vi "Migrate Common Dependencies.vi"(0 "Project path":path, 5 "Measurement path":path, 7 "Dependencies path":path[](array[path]), 11 "error in (no error)":errorcluster) -> (4 "Project reference":refnum<vi>, 6 "MeasurementCore reference":refnum<vi>, 8 "Outside items":string[](array[string]), 15 "error out":errorcluster)   [LabVIEW 2021]
uses:
  controls/Library Info.ctl
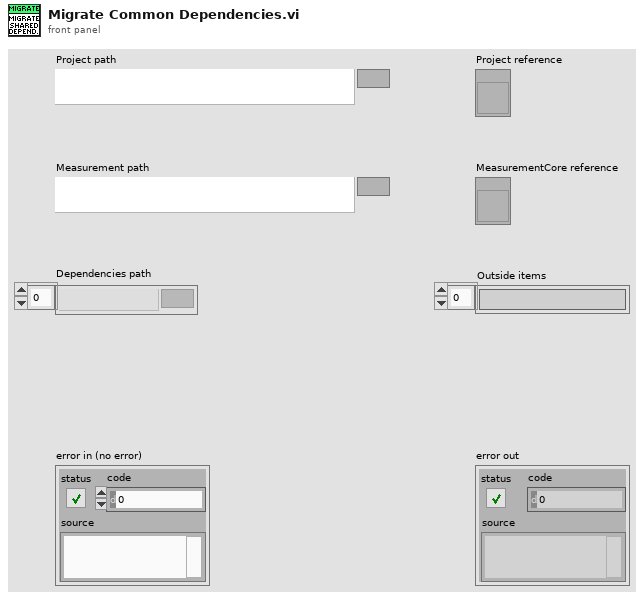
[diagram p1: front panel]
types:
  T1 = typedef "Library Info.ctl" = cluster{"Library path":path, "Library name":string}
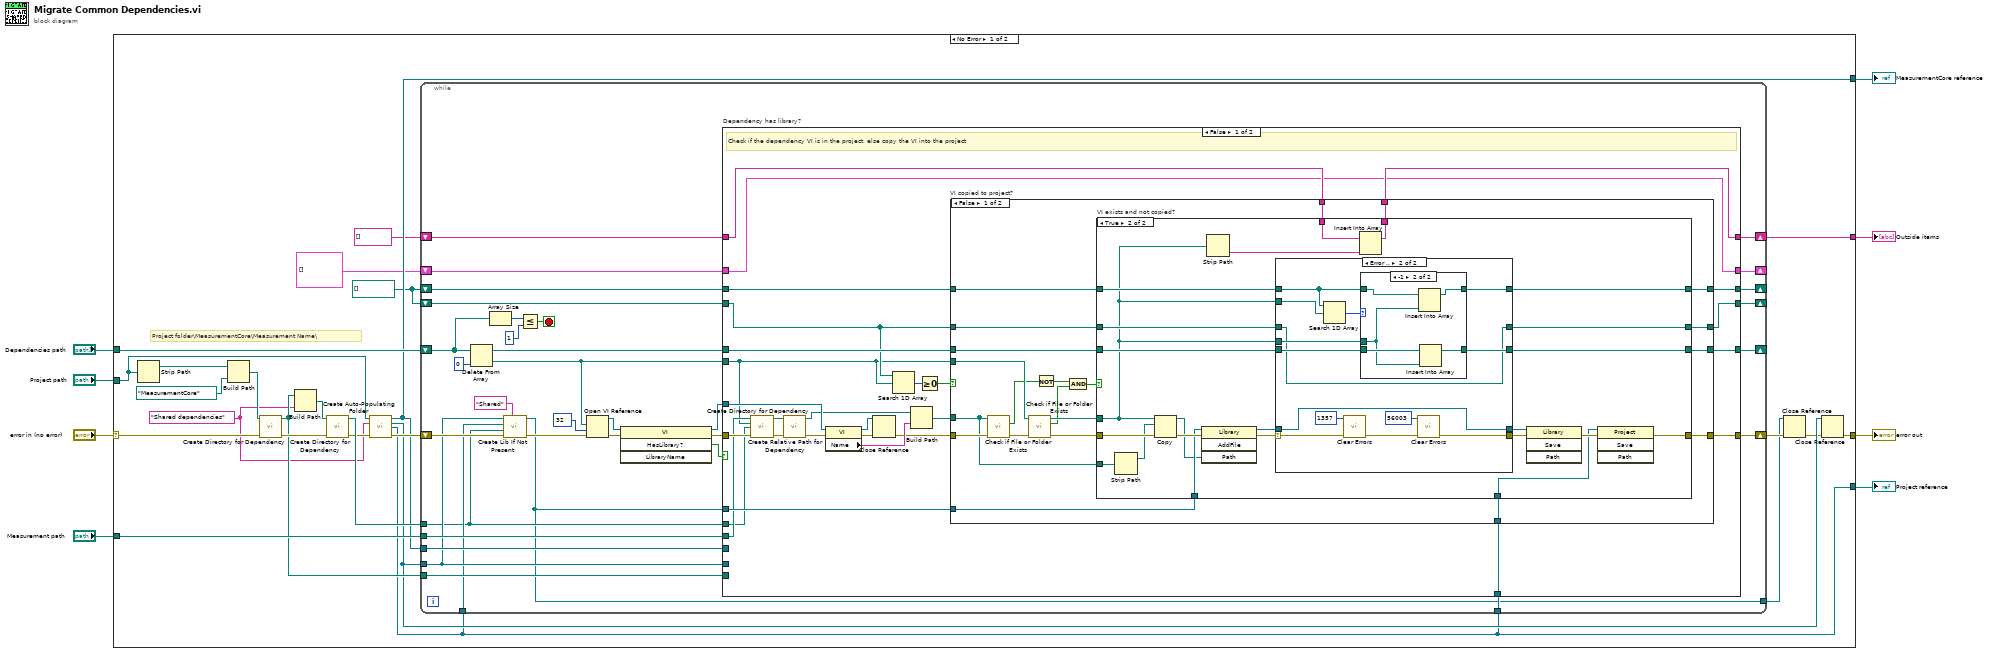
[diagram p0: block diagram]
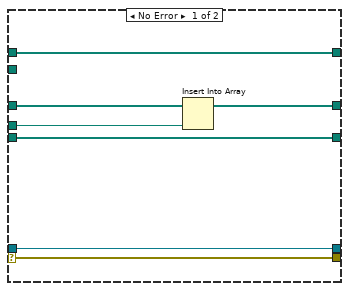
[diagram p3: hidden frame]
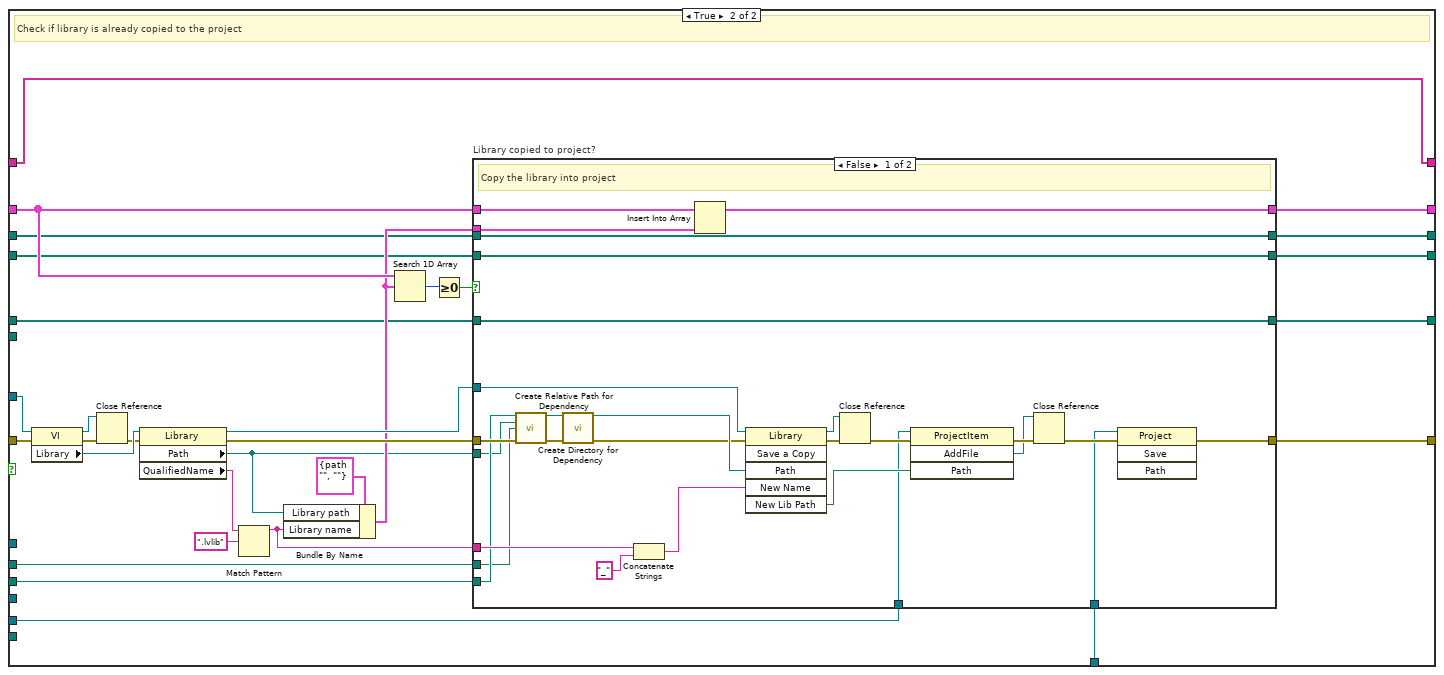
[diagram p6: hidden frame]
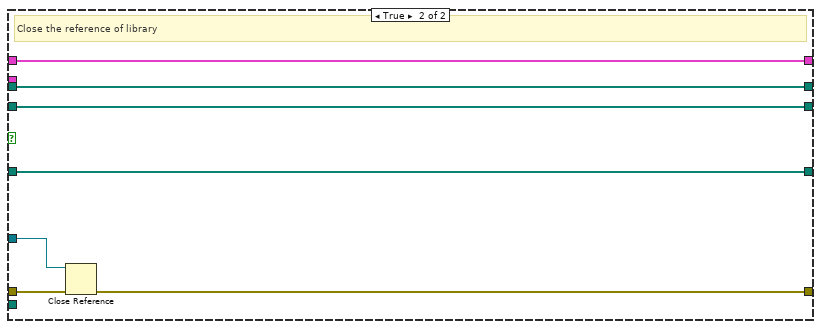
[diagram p7: hidden frame]
diagram:
  n1 = case shown="No Error" "error in (no error)" {
    selector: "error in (no error)" -> [w25 w243]
    tunnel: [w18 w243] -> w7
    tunnel: "Project path" -> [w24 _]
    tunnel: "Measurement path" -> [w29 _]
    tunnel: "Dependencies path" -> [w33 _]
    tunnel: [w20 _] -> w3
    tunnel: [w14 _] -> w2
    tunnel: [w15 _] -> w1
    frame No Error {
      w10 = "Shared dependencies"
      w11 = path[] []
      # "Project folder\\MeasurementCore\\Measurement Name\\"
      n2 = Strip Path(path=w24) -> (stripped path=w28:path)  [unwired: 1 out]
      n3 = Build Path(base path=w28, name or relative path=path "MeasurementCore") -> (appended path=w26:path)
      n4 = call "Create Directory for Dependency.vi"("Directory path"=w26, "error in (no error)"=w25) -> ("Directory path out"=w19:path, "error out"=w23:errorcluster)  [unwired: 12 in]
      n5 = Build Path(base path=w19, name or relative path=w10) -> (appended path=w32:path)
      n6 = call "Create Directory for Dependency.vi"("Directory path"=w32, "error in (no error)"=w23) -> ("Directory path out"=w31:path, "error out"=w22:errorcluster)  [unwired: 12 in]
      n7 = call "Create Auto-Populating Folder.vi"("Project path"=w24, "Plug-in name"=w10, "error in (no error)"=w22) -> ("MeasurementCore reference"=w20:refnum<vi>, "Folder reference"=w17:refnum<vi>, "Project reference"=w14:refnum<vi>, "error out"=w21:errorcluster)  [unwired: 9 in]
      n8 = while {
        shift-right: [w55] -> w30
        shift-left: w21 -> [w43]
        shift-right: [w48] -> _
        shift-left: w33 -> [w65]
        tunnel: w31 -> [w39]
        shift-right: [w54] -> _
        shift-left: T1[] [] -> [w57]
        tunnel: w29 -> [w53]
        shift-right: [w50] -> _
        shift-left: w11 -> [w51]
        tunnel: w20 -> [w47]
        tunnel: w19 -> [w46]
        tunnel: w17 -> [w41]
        shift-right: [w44] -> w15
        shift-left: string[] [] -> [w45]
        tunnel: w14 -> [w40]
        tunnel: w14 -> [w38]
        shift-right: [w37] -> _
        shift-left: w11 -> [w36]
        tunnel: [w35] -> w12
        stop <- w64 stop-if-true
        n9 = Delete From Array(array=w65, index=0) -> (deleted portion=w52:path, array with subset deleted=w49:path[])  [unwired: 1 in]
        n10 = Array Size(array=w65) -> (size(s)=w67:i32)
        n11 = call "Create Lib If Not Present.vi"("Plug-in name"="Shared", "error in (no error)"=w43, "DestDirectory"=w39, "ProjectRef"=w40, "VirtualFolderRef"=w41) -> ("error out"=w42:errorcluster, "Library Refnum"=w35:refnum<vi>)  [unwired: 5 in]
        n12 = Less Or Equal?(x=w67, y=1) -> (x <= y?=w64:bool)
        n13 = Open VI Reference(vi path=w52, options=32, error in (no error)=w42) -> (vi reference=w61:refnum<vi>, error out=w63:errorcluster)  [unwired: 3 in]
        n14 = invoke class="VI" method="HasLibrary?"(reference=w61, error in=w63) -> (reference out=w58:refnum<vi>, error out=w59:errorcluster, "Has Library?"=w60:bool)  [unwired: 2 in, 1 out]
        n15 = case "Dependency has library?" shown="False" w60 {
          tunnel: w59 -> [w73 w206]
          tunnel: w58 -> [w94 w207]
          tunnel: w57 -> [w77 w194]
          tunnel: [w89 w195] -> w55
          tunnel: [w77 w193] -> w54
          tunnel: w53 -> [w72 w191]
          tunnel: w39 -> [w70 w189]
          tunnel: w52 -> [w71 _]
          tunnel: w51 -> [w85 w186]
          tunnel: [w81 w185] -> w50
          tunnel: w49 -> [w88 w184]
          tunnel: [w87 w183] -> w48
          tunnel: w47 -> [_ _]
          tunnel: w46 -> [_ _]
          tunnel: w41 -> [_ w182]
          tunnel: w45 -> [w79 w181]
          tunnel: [w78 w181] -> w44
          tunnel: w35 -> [w80 _]
          tunnel: w38 -> [w74 w180]
          tunnel: [w76 w178] -> w37
          tunnel: w36 -> [w75 w179]
          frame False {
            # "Check if the dependency VI is in the project, else copy the VI into the project"
            n16 = call "Create Relative Path for Dependency.vi"("Old Main Path"=w72, "Old Dependency Path"=w71, "New Dir"=w70, "error in (no error)"=w73) -> ("Directory"=w68:path, "error out"=w69:errorcluster)  [unwired: 10 in]
            n17 = call "Create Directory for Dependency.vi"("Directory path"=w68, "error in (no error)"=w69) -> ("Directory path out"=w86:path, "error out"=w95:errorcluster)  [unwired: 12 in]
            n18 = property class="VI"(reference=w94, error in=w95) -> (reference out=w90:refnum<vi>, error out=w93:errorcluster, "Name"=w92:string)
            n19 = Close Reference(reference=w90, error in (no error)=w93) -> (error out=w91:errorcluster)
            n20 = Search 1D Array(1D array=w85, element=w71) -> (index of element=w84:i32)  [unwired: 1 in]
            n21 = Build Path(base path=w86, name or relative path=w92) -> (appended path=w83:path)
            n22 = Greater Or Equal To 0?(x=w84) -> (x >= 0?=w82:bool)
            n23 = case "VI copied to project?" shown="False" w82 {
              tunnel: w91 -> [w116 w177]
              tunnel: w71 -> [w115 _]
              tunnel: [w112 w177] -> w89
              tunnel: w85 -> [w111 w176]
              tunnel: [w110 w176] -> w81
              tunnel: w83 -> [w106 _]
              tunnel: w88 -> [w109 w175]
              tunnel: [w108 w175] -> w87
              tunnel: w79 -> [w101 w174]
              tunnel: [w100 w174] -> w78
              tunnel: w80 -> [w99 _]
              tunnel: [w98 w173] -> w76
              tunnel: w75 -> [w97 w173]
              tunnel: w74 -> [w96 _]
              frame False {
                n24 = call <vilib>:"Check if File or Folder Exists.vi"("error in (no error)"=w116, "path"=w106) -> ("error out"=w107:errorcluster, "file or folder exists?"=w105:bool)  [unwired: 7 in, 1 out]
                n25 = call <vilib>:"Check if File or Folder Exists.vi"("error in (no error)"=w107, "path"=w115) -> ("error out"=w114:errorcluster, "file or folder exists?"=w103:bool, "dup path"=w113:path)  [unwired: 7 in]
                n26 = Not(x=w105) -> (.not. x?=w104:bool)
                n27 = And(x=w104, y=w103) -> (x .and. y?=w102:bool)
                n28 = case "VI exists and not copied?" shown="True" w102 {
                  tunnel: w114 -> [w121 w144]
                  tunnel: w113 -> [_ w122]
                  tunnel: [w121 w124] -> w112
                  tunnel: w111 -> [w120 w143]
                  tunnel: [w120 w142] -> w110
                  tunnel: w106 -> [_ w138]
                  tunnel: w109 -> [w119 w126]
                  tunnel: [w119 w125] -> w108
                  tunnel: w101 -> [w118 w137]
                  tunnel: [w118 w135] -> w100
                  tunnel: w99 -> [_ w134]
                  tunnel: [w117 w132] -> w98
                  tunnel: w97 -> [w117 w131]
                  tunnel: w96 -> [_ w123]
                  frame False {
                  }
                  frame True {
                    n29 = Strip Path(path=w138) -> (stripped path=w140:path)  [unwired: 1 out]
                    n30 = Copy(8:w144, 10:w140, 11:w122) -> (0:w141:errorcluster, 3:w133:path)  [unwired: 2 in, 1 out]
                    n31 = invoke class="Library" method="AddFile"(reference=w134, error in=w141, "Path"=w133) -> (reference out=w130:refnum<vi>, error out=w129:errorcluster)  [unwired: 1 in, 2 out]
                    n32 = Strip Path(path=w122) -> (name=w136:string)  [unwired: 1 out]
                    n33 = case shown="Error .." w129 {
                      selector: w129 -> [w146 w165]
                      tunnel: w143 -> [w151 w152]
                      tunnel: [w150 w152] -> w142
                      tunnel: w122 -> [w149 w155]
                      tunnel: [w148 w156] -> w132
                      tunnel: w131 -> [w148 w157]
                      tunnel: [w147 w154] -> w127
                      tunnel: w130 -> [w147 w154]
                      tunnel: [w146 w163] -> w128
                      tunnel: w126 -> [w145 w159]
                      tunnel: [w145 w158] -> w125
                      tunnel: w122 -> [_ w160]
                      frame No Error {
                        n34 = Insert Into Array(array=w151, new element=w149) -> (w150:path[])  [unwired: 1 in]
                      }
                      frame Error {
                        n35 = Search 1D Array(1D array=w157, element=w160) -> (index of element=w153:i32)  [unwired: 1 in]
                        n36 = call <vilib>:"Clear Errors.vi"("error in (no error)"=w165, "specific error code to clear (0: all)"=1357) -> ("error out"=w164:errorcluster)  [unwired: 4 in, 1 out]
                        n37 = case shown="-1" w153 {
                          tunnel: w159 -> [w166 w172]
                          tunnel: [w166 w171] -> w158
                          tunnel: w157 -> [w167 w170]
                          tunnel: [w167 w169] -> w156
                          tunnel: w155 -> [_ w168]
                          frame Default {
                          }
                          frame -1 {
                            n38 = Insert Into Array(array=w170, new element=w168) -> (w169:path[])  [unwired: 1 in]
                            n39 = Insert Into Array(array=w172, new element=w168) -> (w171:path[])  [unwired: 1 in]
                          }
                        }
                        n40 = call <vilib>:"Clear Errors.vi"("error in (no error)"=w164, "specific error code to clear (0: all)"=56003) -> ("error out"=w163:errorcluster)  [unwired: 4 in, 1 out]
                      }
                    }
                    n41 = Insert Into Array(array=w137, new element=w136) -> (w135:string[])  [unwired: 1 in]
                    n42 = invoke class="Library" method="Save"(reference=w127, error in=w128) -> (error out=w139:errorcluster)  [unwired: 2 in, 3 out]
                    n43 = invoke class="Project" method="Save"(reference=w123, error in=w139) -> (error out=w124:errorcluster)  [unwired: 2 in, 3 out]
                  }
                }
              }
              frame True {
              }
            }
          }
          frame True {
            # "Check if library is already copied to the project"
            n44 = property class="VI"(reference=w207, error in=w206) -> (reference out=w197:refnum<vi>, error out=w205:errorcluster, "Library"=w204:refnum<vi>)
            n45 = Close Reference(reference=w197, error in (no error)=w205) -> (error out=w198:errorcluster)
            n46 = property class="Library"(reference=w204, error in=w198) -> (reference out=w196:refnum<vi>, error out=w199:errorcluster, "Path"=w190:path, "QualifiedName"=w200:string)
            n47 = Match Pattern(string=w200, regular expression=".lvlib") -> (before substring=w187:string)  [unwired: 1 in, 3 out]
            n48 = Bundle By Name(cluster=T1 {"Library path"=path "", "Library name"=""} ("Cluster"), "Library path"=w190, "Library name"=w187) -> (w192:T1)
            n49 = Search 1D Array(1D array=w194, element=w192) -> (index of element=w202:i32)  [unwired: 1 in]
            n50 = Greater Or Equal To 0?(x=w202) -> (x >= 0?=w201:bool)
            n51 = case "Library copied to project?" shown="False" w201 {
              tunnel: w199 -> [w212 w241]
              tunnel: w196 -> [w229 w242]
              tunnel: [w216 w240] -> w195
              tunnel: w194 -> [w235 w239]
              tunnel: [w234 w239] -> w193
              tunnel: w192 -> [w233 _]
              tunnel: w191 -> [w211 _]
              tunnel: w190 -> [w210 _]
              tunnel: w189 -> [w209 _]
              tunnel: w187 -> [w219 _]
              tunnel: w186 -> [w226 w238]
              tunnel: [w226 w238] -> w185
              tunnel: [w225 w237] -> w183
              tunnel: w184 -> [w225 w237]
              tunnel: w182 -> [w220 _]
              tunnel: w180 -> [w215 _]
              tunnel: [w214 w236] -> w178
              tunnel: w179 -> [w214 w236]
              frame False {
                # "Copy the library into project"
                n52 = call "Create Relative Path for Dependency.vi"("Old Main Path"=w211, "Old Dependency Path"=w210, "New Dir"=w209, "error in (no error)"=w212) -> ("Directory"=w208:path, "error out"=w213:errorcluster)  [unwired: 10 in]
                n53 = call "Create Directory for Dependency.vi"("Directory path"=w208, "error in (no error)"=w213) -> ("Directory path out"=w230:path, "error out"=w228:errorcluster)  [unwired: 12 in]
                n54 = Concatenate Strings(w219, "_" ("string")) -> (w217:string)
                n55 = Insert Into Array(array=w235, new element=w233) -> (w234:T1[])  [unwired: 1 in]
                n56 = invoke class="Library" method="Save a Copy"(reference=w229, error in=w228, "Path"=w230, "New Name"=w217) -> (reference out=w231:refnum<vi>, error out=w232:errorcluster, "New Lib Path"=w223:path)  [unwired: 2 in, 3 out]
                n57 = Close Reference(reference=w231, error in (no error)=w232) -> (error out=w227:errorcluster)
                n58 = invoke class="ProjectItem" method="AddFile"(reference=w220, error in=w227, "Path"=w223) -> (error out=w224:errorcluster, "AddFile"=w221:refnum<vi>)  [unwired: 1 in, 2 out]
                n59 = Close Reference(reference=w221, error in (no error)=w224) -> (error out=w222:errorcluster)
                n60 = invoke class="Project" method="Save"(reference=w215, error in=w222) -> (error out=w216:errorcluster)  [unwired: 2 in, 3 out]
              }
              frame True {
                # "Close the reference of library"
                n61 = Close Reference(reference=w242, error in (no error)=w241) -> (error out=w240:errorcluster)
              }
            }
          }
        }
      }
      n62 = Close Reference(reference=w12, error in (no error)=w30) -> (error out=w13:errorcluster)
      n63 = Close Reference(reference=w17, error in (no error)=w13) -> (error out=w18:errorcluster)
    }
    frame Error {
    }
  }
  "error out" <- w7
  "MeasurementCore reference" <- w3
  "Project reference" <- w2
  "Outside items" <- w1
